vi "Config Mods.vi"(8 "error in (no error)":errorcluster, 10 "ECAT Mod Reconfig in":T1[](array[typedef]), 11 "RSI Modules in":T2[](array[typedef]) {"Module Config Data"."Config Block Data Refs"."Data Reference" format="%.0x"; "CDOutput Data"."BD Refs"."Data Reference" format="%.0x"; "CDInput Data"."BD Refs"."Data Reference" format="%.0x"; "VS ref" format="%.0x"}) -> (0 "error out":errorcluster, 2 "ECAT Mod Reconfig out":T1[](array[typedef]), 3 "RSI Modules out":T2[](array[typedef]) {"Module Config Data"."Config Block Data Refs"."Data Reference" format="%.0x"; "CDOutput Data"."BD Refs"."Data Reference" format="%.0x"; "CDInput Data"."BD Refs"."Data Reference" format="%.0x"; "VS ref" format="%.0x"})   [LabVIEW 2019, in "SEECD Engine.lvlib"]
uses:
  SEECD Engine.lvlib
  Type Defs/RSI Module Data.ctl
  <vilib>/NI VeriStand/Custom Device API/Custom Device Item Ref.ctl
  Type Defs/Open Module IOVs.ctl
  Modules.lvlibp/RSI Module/RSI Module.lvclass
  Modules.lvlibp/RSI Module/Module Models.ctl
  Modules.lvlibp/RSI Module/Channel Type.ctl
  Type Defs/Input Data.ctl
  <vilib>/NI VeriStand/Custom Device API/Block Data Reference.ctl
  <vilib>/NI VeriStand/Custom Device API/Data Reference.ctl
  Type Defs/Output Data.ctl
  Type Defs/Module Config Data.ctl
  Type Defs/Mixed IO.ctl
  Type Defs/ECAT Module Reconfig.ctl
  <vilib>/NI VeriStand/Custom Device API/Custom Device API.lvlib
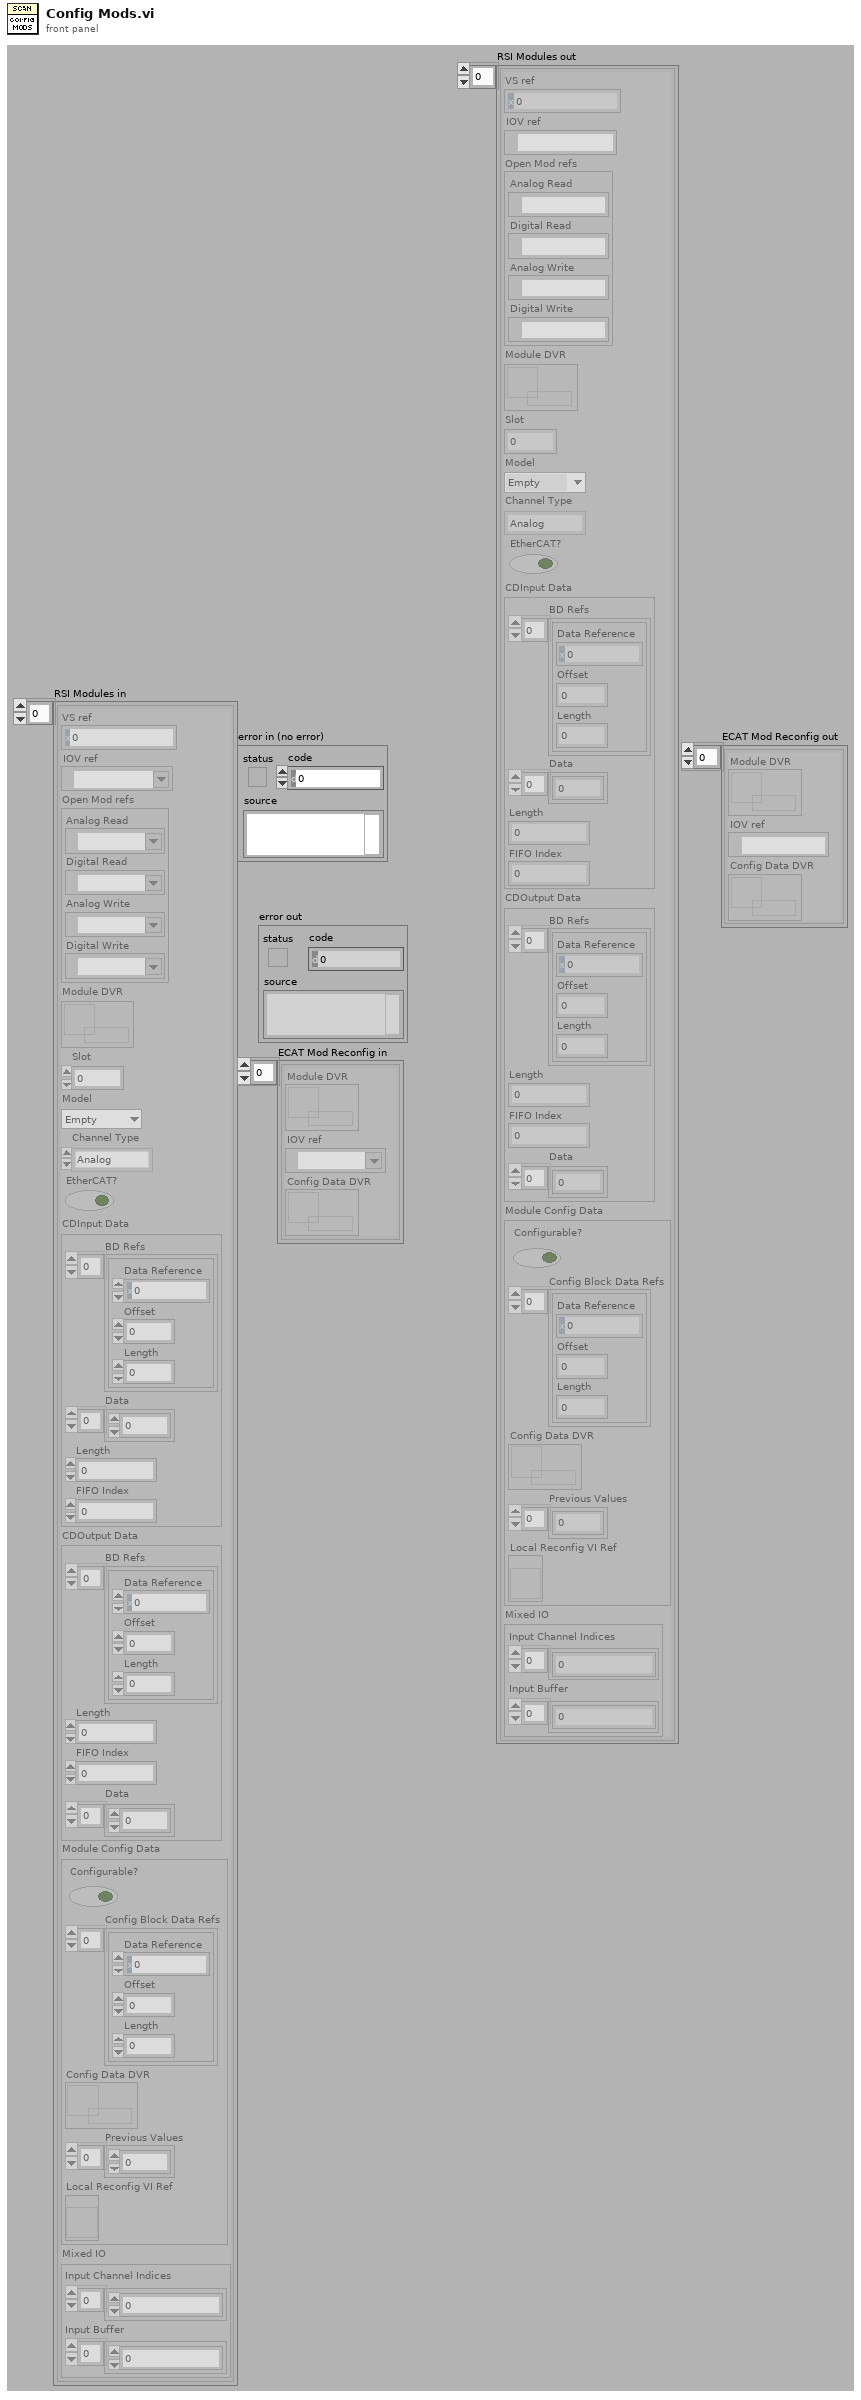
[diagram p1: front panel]
types:
  T1 = typedef "SEECD Engine.lvlib/ECAT Module Reconfig.ctl" = cluster{"Module DVR":refnum<data-value>, "IOV ref":refnum<k21>, "Config Data DVR":refnum<data-value>}
  T2 = typedef "SEECD Engine.lvlib/RSI Module Data.ctl" = cluster{"VS ref":T3, "IOV ref":refnum<k21>, "Open Mod refs":T4, "Module DVR":refnum<data-value>, "Slot":u32, "Model":T5, "Channel Type":T6, "EtherCAT?":bool, "CDInput Data":T7, "CDOutput Data":T10, "Module Config Data":T11, "Mixed IO":T12}
  T3 = typedef "Custom Device API.lvlib/Custom Device Item Ref.ctl" = u64
  T4 = typedef "SEECD Engine.lvlib/Open Module IOVs.ctl" = cluster{"Analog Read":refnum<k21>, "Digital Read":refnum<k21>, "Analog Write":refnum<k21>, "Digital Write":refnum<k21>}
  T5 = typedef "Modules.lvlibp/RSI Module.lvclass/Module Models.ctl" = enum16{"Empty", "NI 9201", "NI 9203", "NI 9205", "NI 9206", "NI 9207", "NI 9208", "NI 9209", "NI 9210", "NI 9211", "NI 9212", "NI 9213", "NI 9214", "NI 9215", "NI 9216", "NI 9217", "NI 9219", "NI 9220", "NI 9221", "NI 9222", "NI 9223", "NI 9224", "NI 9225", "NI 9226", "NI 9227", "NI 9228", "NI 9229", "NI 9233", "NI 9234", "NI 9235", "NI 9236", "NI 9237", "NI 9239", "NI 9242", "NI 9244", "NI 9253", "NI 9263", "NI 9264", "NI 9265", "NI 9266", "NI 9269", "NI 9344", "NI 9350", "NI 9375", "NI 9401", "NI 9402", "NI 9403", "NI 9411", "NI 9421", "NI 9422", "NI 9423", "NI 9425", "NI 9426", "NI 9435", "NI 9436", "NI 9437", "NI 9472", "NI 9474", "NI 9475", "NI 9476", "NI 9477", "NI 9478", "NI 9481", "NI 9482", "NI 9485"}
  T6 = typedef "Modules.lvlibp/RSI Module.lvclass/Channel Type.ctl" = enum16{"Analog", "Digital"}
  T7 = typedef "SEECD Engine.lvlib/Input Data.ctl" = cluster{"BD Refs":T8[], "Data":dbl[], "Length":i32, "FIFO Index":i32}
  T8 = typedef "Custom Device API.lvlib/Block Data Reference.ctl" = cluster{"Data Reference":T9, "Offset":u64, "Length":u64}
  T9 = typedef "Custom Device API.lvlib/Data Reference.ctl" = i32
  T10 = typedef "SEECD Engine.lvlib/Output Data.ctl" = cluster{"BD Refs":T8[], "Length":i32, "FIFO Index":i32, "Data":dbl[]}
  T11 = typedef "SEECD Engine.lvlib/Module Config Data.ctl" = cluster{"Configurable?":bool, "Config Block Data Refs":T8[], "Config Data DVR":refnum<data-value>, "Previous Values":dbl[], "Local Reconfig VI Ref":refnum<vi>}
  T12 = typedef "SEECD Engine.lvlib/Mixed IO.ctl" = cluster{"Input Channel Indices":i32[], "Input Buffer":dbl[]}
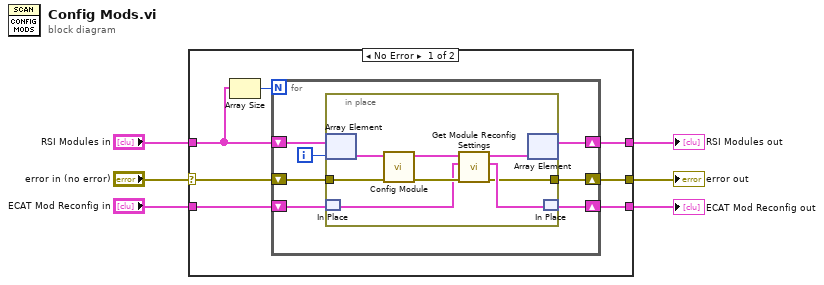
[diagram p0: block diagram]
diagram:
  n1 = case shown="No Error" "error in (no error)" {
    selector: "error in (no error)" -> [w7 w31]
    tunnel: "RSI Modules in" -> [w12 w30]
    tunnel: [w11 w30] -> w5
    tunnel: [w10 w31] -> w4
    tunnel: "ECAT Mod Reconfig in" -> [w9 w29]
    tunnel: [w8 w29] -> w2
    frame No Error {
      n2 = Array Size(array=w12) -> (size(s)=w13:i32)
      n3 = for {
        N: w13 -> [_]
        shift-right: [w16] -> w10
        shift-left: w7 -> [w18]
        shift-right: [w17] -> w11
        shift-left: w12 -> [w20]
        shift-right: [w14] -> w8
        shift-left: w9 -> [w15]
        i -> [w19]
        n4 = in-place {
          in-place-border: w18 -> [w27]
          in-place-border: [w21] -> w16
          n5 = in-place-array #1(w20, w19) -> (w28:T2)
          n6 = in-place-match #2(w15) -> (w24:T1[])
          n7 = call "Config Module.vi"("error in (no error)"=w27, "RSI Module in"=w28) -> ("error out"=w25:errorcluster, "RSI Module out"=w26:T2)  [unwired: 8 in]
          n8 = call "Get Module Reconfig Settings.vi"("error in (no error)"=w25, "ECAT Mod Reconfig in"=w24, "RSI Module in"=w26) -> ("error out"=w21:errorcluster, "ECAT Mod Reconfig out"=w23:T1[], "RSI Module out"=w22:T2)  [unwired: 6 in]
          n9 = in-place-array #1(w22) -> (w17:T2[])  [unwired: 1 out]
          n10 = in-place-match #2(w23) -> (w14:T1[])
        }
      }
    }
    frame Error {
    }
  }
  "RSI Modules out" <- w5
  "error out" <- w4
  "ECAT Mod Reconfig out" <- w2
